vi "2HP_EnFlo_Specific - USB.vi"(5 "Datalog file path (full)":path, 6 "COM port":refnum<visa-resource-name>, 7 "Log data stream":bool, 8 "Set data rate (Hz)":u8(ring)=14 items=["1", "2", "4", "5", "8", "10", "16", "20", "25", "32", "40", "50", "64", "80", "100", "125", "160", "200", "250", "320", "400", "500", "625", "800", "1000"], 9 "N samples":u32=1000, 10 "Command":T2="s") -> (0 "Error":errorcluster, 2 "All samples out":sgl[][](array[numeric]), 3 "Rendezvous out":bool)   [LabVIEW 2020]
uses:
  ctls/2HP_Cmd (USB).ctl
  Globals/Meas_global.vi
panel:
  in  "Main":T1(tab)
  out "Serial number":u32 format="%0d"
  out "Pressure sensor EEPROM checksums ok":bool[](array[boolean])
  out "Pressure sensor temperatures in range":bool[](array[boolean])
  out "Pressure sensor values in range":bool[](array[boolean])
  out "Subsystems ok":bool[](array[boolean])
  out "n":u16
  out "Auto zero progBar":u16(slide) caption="Collecting samples, please maintain dP = 0" scale=0.0..1000.0
  out "P_raw_Azero":sgl[](array[numeric])
  in  "EEPROM array":sgl[](array[numeric])
  out "Chk ok":bool
  out "EEPROM CRC16":u16 format="%04x"
  out "received":bool
  out "Returned data rate (Hz)":u16
  out "sent":bool
  out "frm err":u32
  out "chk err":u32
  in  "Stop Data":bool
  out "Relative humidity (%)":sgl
  out "Env. sensor die temperature (deg C)":sgl
  out "External thermistor temperature (deg C)":sgl
  out "Atmospheric pressure (mbar)":sgl
  out "Checksum ok":bool
  out "Gyration vector (deg / s)":sgl[](array[numeric])
  out "Acceleration vector (g)":sgl[](array[numeric])
  out "Pressures":sgl[][](graph)
  out "Stream enabled":bool
  # "Paul Nathan 10/2020"
  # "Output array order:\nP0.... (Pa)\nP1.... (Pa)\nP_atmos (mbar)....\nT_ext (deg C)....\nT_env (deg C)....\nRH (%)....\nax (g)....\nay (g)....\naz (g)....\nwx (deg / s)....\nwy (deg / s)....\nwz (deg / s)...."
  # "Pressure sensor 0 EEPROM checksum okay"
  # "Pressure sensor 1 EEPROM checksum okay"
  # "Pressure sensor 0 temperature in range"
  # "Pressure sensor 1 temperature in range"
  # "Pressure sensor 0 value in range"
  # "Pressure sensor 1 value in range"
  # "Environmental sensor present"
  # "Inertial sensor present"
  # "Accelerometer self test pass"
  # "Gyroscope self test pass"
  # "External thermistor value in range"
  # "MCU EEPROM checksum ok"
  # "of 1000"
  # "P0 raw auto-zero"
  # "P1 raw auto-zero"
  # "P0 raw auto-zero"
  # "P1 raw auto-zero"
  # "Atmospheric pressure offset (Pa)"
  # "External thermistor temperature offset (deg C)"
  # "Serial number"
  # "RS-485 baud rate (bps)"
  # "Accelerometer vector magnitude scale factor"
  # "(reserved, 0x00000000)"
  # "(reserved, 0x00000000)"
  # "Gyroscope x component offset (deg / s)"
  # "Gyroscope y component offset (deg / s)"
  # "Gyroscope z component offset (deg / s)"
  # "RS-485 address"
  # "w_x"
  # "w_y"
  # "w_z"
  # "a_x"
  # "a_y"
  # "a_z"
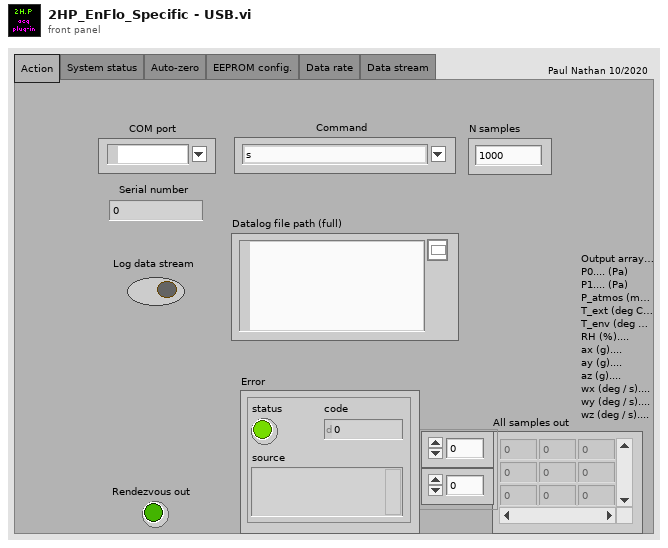
[diagram p1: front panel]
types:
  T1 = enum32{"Action", "System status", "Auto-zero", "EEPROM config.", "Data rate", "Data stream"}
  T2 = typedef "2HP_Cmd (USB).ctl" = string
  T3 = enum16{"open", "replace", "create", "open or create", "replace or create", "replace or create with confirmation"}
  T4 = typedef "Rendezvous RefNum" = refnum<k1>
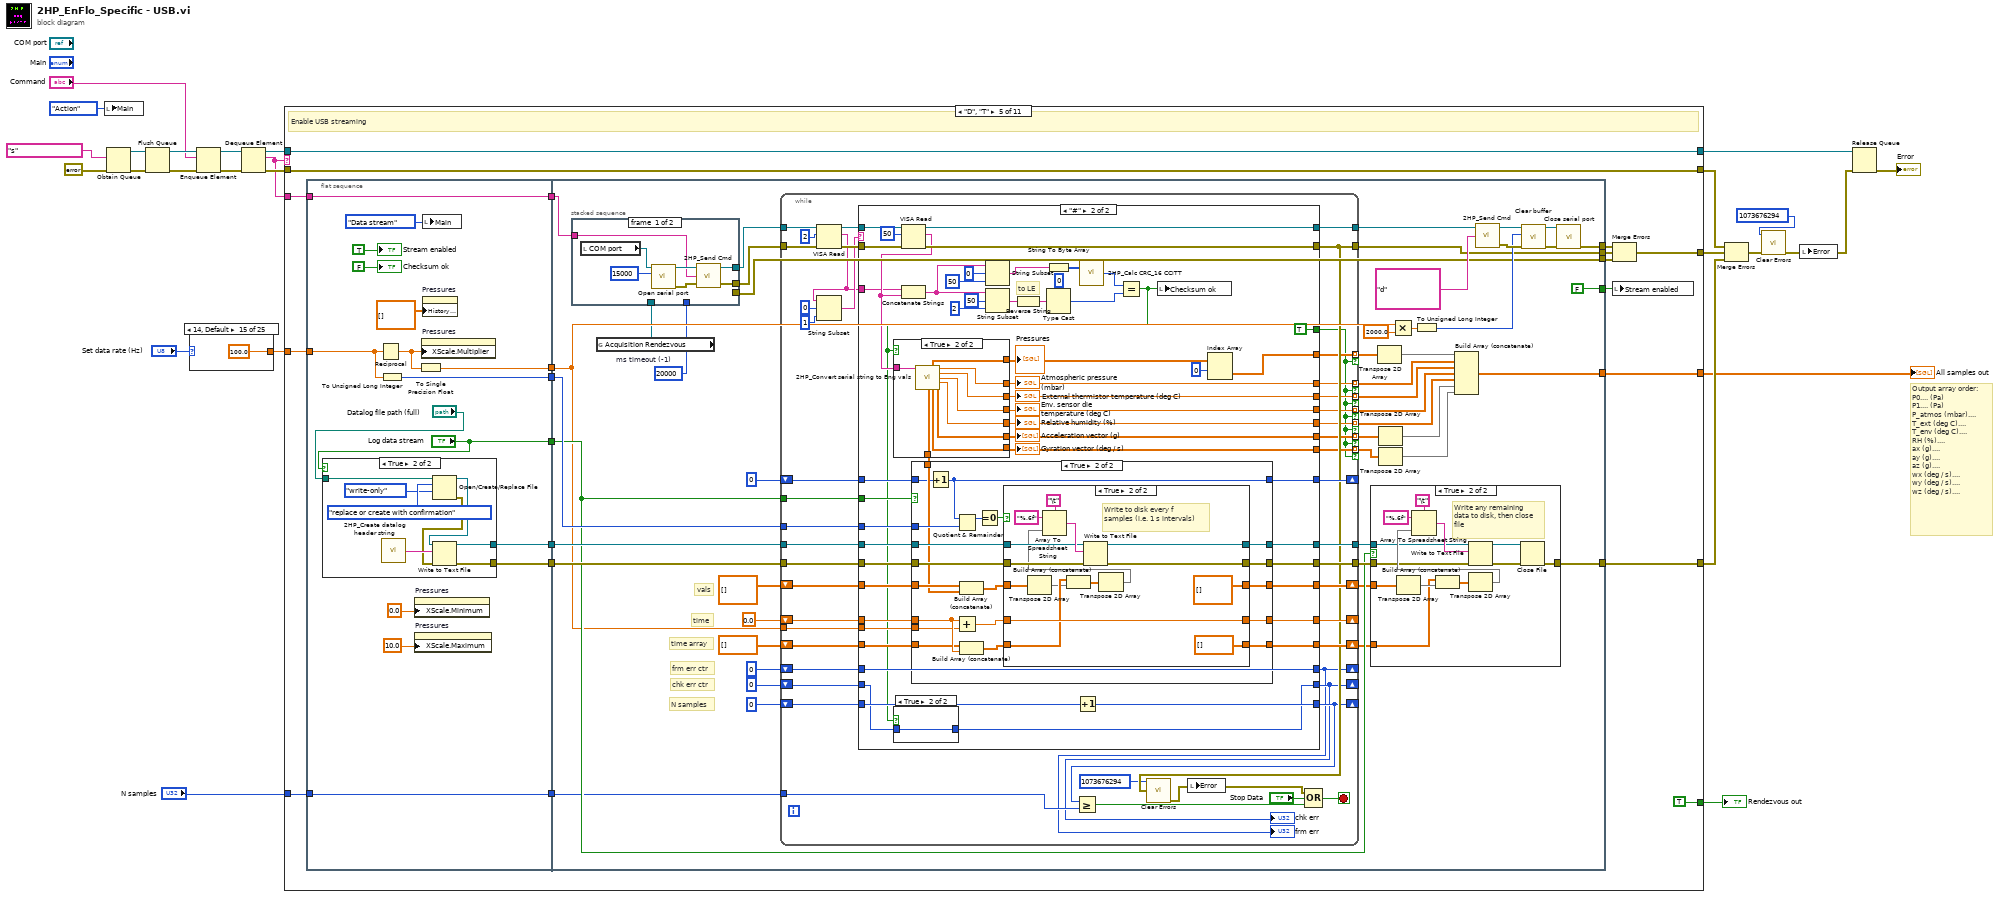
[diagram p0: block diagram]
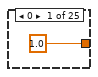
[diagram p2: hidden frame]
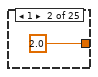
[diagram p3: hidden frame]
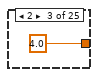
[diagram p4: hidden frame]
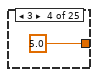
[diagram p5: hidden frame]
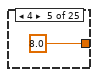
[diagram p6: hidden frame]
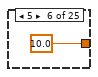
[diagram p7: hidden frame]
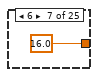
[diagram p8: hidden frame]
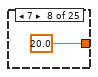
[diagram p9: hidden frame]
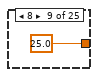
[diagram p10: hidden frame]
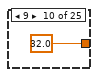
[diagram p11: hidden frame]
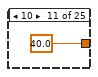
[diagram p12: hidden frame]
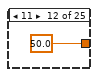
[diagram p13: hidden frame]
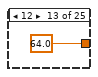
[diagram p14: hidden frame]
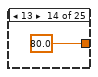
[diagram p15: hidden frame]
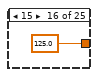
[diagram p16: hidden frame]
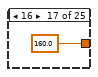
[diagram p17: hidden frame]
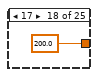
[diagram p18: hidden frame]
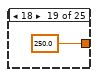
[diagram p19: hidden frame]
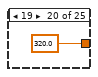
[diagram p20: hidden frame]
diagram:
  # "Output array order:\nP0.... (Pa)\nP1.... (Pa)\nP_atmos (mbar)....\nT_ext (deg C)....\nT_env (deg C)....\nRH (%)....\nax (g)....\nay (g)....\naz (g)....\nwx (deg / s)....\nwy (deg / s)....\nwz (deg / s)...."
  n1 = local write "Main"(T1."Action" ("Main")) -> ()
  n2 = Obtain Queue(element data type=T2 "s" ("Combo Box"), error in (no error)=errorcluster {"status"=FALSE, "code"=0, "source"=""}) -> (queue out=w24:refnum<queue>, error out=w25:errorcluster)  [unwired: 3 in, 1 out]
  n3 = Flush Queue(queue=w24, error in (no error)=w25) -> (queue out=w23:refnum<queue>, error out=w18:errorcluster)  [unwired: 1 out]
  n4 = case shown="14, Default" "Set data rate (Hz)" {
    tunnel: [1.0 2.0 4.0 5.0 8.0 10.0 16.0 20.0 25.0 32.0 40.0 50.0 64.0 80.0 100.0 125.0 160.0 200.0 250.0 320.0 400.0 500.0 625.0 800.0 1000.0] -> w3
    frame 0 {
    }
    frame 1 {
    }
    frame 2 {
    }
    frame 3 {
    }
    frame 4 {
    }
    frame 5 {
    }
    frame 6 {
    }
    frame 7 {
    }
    frame 8 {
    }
    frame 9 {
    }
    frame 10 {
    }
    frame 11 {
    }
    frame 12 {
    }
    frame 13 {
    }
    frame 14, Default {
    }
    frame 15 {
    }
    frame 16 {
    }
    frame 17 {
    }
    frame 18 {
    }
    frame 19 {
    }
    frame 20 {
    }
    frame 21 {
    }
    frame 22 {
    }
    frame 23 {
    }
    frame 24 {
    }
  }
  n5 = Enqueue Element(queue=w23, element="Command", error in (no error)=w18) -> (queue out=w19:refnum<queue>, error out=w17:errorcluster)  [unwired: 1 in, 1 out]
  n6 = Dequeue Element(queue=w19, error in (no error)=w17) -> (queue out=w14:refnum<queue>, element=w12:T2, error out=w13:errorcluster)  [unwired: 1 in, 1 out]
  n7 = case shown="\"D\", \"T\"" w12 {
    tunnel: w14 -> [w57 w96 w133 w183 w237 w518 w542 w596 w629 w652 w656]
    tunnel: [w57 w96 w133 w183 w237 w518 w542 w596 w629 w652 w656] -> w15
    tunnel: w13 -> [w56 w95 w132 w182 w236 w517 w543 w597 w628 w651 w655]
    tunnel: [w56 w95 w132 w182 w236 w517 w543 w597 w628 w651 w655] -> w11
    tunnel: w12 -> [w55 w94 w131 w181 w235 w520 w545 w599 w627 _ _]
    tunnel: [w53 w92 w129 w179 w220 w519 w544 w598 w625 errorcluster {"status"=FALSE, "code"=0, "source"=""} ("Error out") errorcluster {"status"=FALSE, "code"=0, "source"=""} ("Error out")] -> w10
    tunnel: [_ _ _ _ w233 _ _ _ _ _ _] -> w9
    tunnel: "N samples" -> [_ _ _ _ w226 _ _ _ _ _ _]
    tunnel: [_ _ _ _ w224 _ _ _ _ _ _] -> w5
    tunnel: w3 -> [_ _ _ _ w223 w515 _ _ _ _ _]
    tunnel: [FALSE FALSE FALSE FALSE TRUE FALSE FALSE FALSE FALSE FALSE FALSE] -> w1
    frame "S", "s" {
      # "Perform self-test and retrieve status bytes, Retrieve status bytes"
      n8 = flat-sequence {
        tunnel: w55 -> [w60]
        tunnel: [w60] -> w54
        tunnel: w54 -> [w66]
        tunnel: [w61] -> w53
        frame #0 {
          w59 = bool[] [] ("Pressure sensor EEPROM checksums ok")
          n9 = local write "Main"(T1."System status" ("Main")) -> ()
          "Pressure sensor EEPROM checksums ok" <- w59
          "Pressure sensor temperatures in range" <- w59
          "Pressure sensor values in range" <- w59
          "Subsystems ok" <- w59
        }
        frame #1 {
          w70 = 1 ("length (rest)")
          w78 = u8 0 ("byte count")
          n10 = local read "COM port"() -> (w67:refnum<visa-resource-name>)
          n11 = call "Open serial port.vi"("timeout (ms)"=u32 5000, "VISA resource name"=w67) -> ("Error out"=w88:errorcluster, "VISA resource name out"=w89:refnum<visa-resource-name>)  [unwired: 8 in]
          n12 = call "2HP_Send Cmd.vi"("Error In"=w88, "Operation"=w66, "Port"=w89) -> ("Error Out"=w86:errorcluster, "Port out"=w87:refnum<visa-resource-name>)  [unwired: 1 in]
          n13 = VISA Read(VISA resource name=w87, byte count=u32 4, error in (no error)=w86) -> (VISA resource name out=w84:refnum<visa-resource-name>, read buffer=w73:string, error out=w83:errorcluster)  [unwired: 1 out]
          n14 = call "Close serial port.vi"("Error in"=w83, "VISA resource name"=w84) -> ("Error out"=w61:errorcluster)  [unwired: 9 in]
          n15 = String Subset(string=w73, offset (0)=0, length (rest)=w70) -> (substring=w82:string)
          n16 = String Subset(string=w73, offset (0)=1, length (rest)=w70) -> (substring=w81:string)
          n17 = String Subset(string=w73, offset (0)=2 ("length (rest)"), length (rest)=w70) -> (substring=w80:string)
          n18 = String Subset(string=w73, offset (0)=3, length (rest)=w70) -> (substring=w79:string)
          n19 = Type Cast(type=w78, x=w82) -> (*(type *) &x=w77:u8)
          n20 = Type Cast(type=w78, x=w81) -> (*(type *) &x=w76:u8)
          n21 = Type Cast(type=w78, x=w80) -> (*(type *) &x=w75:u8)
          n22 = Type Cast(type=w78, x=w79) -> (*(type *) &x=w74:u8)
          n23 = Number To Boolean Array(number=w77) -> (Boolean array=w65:bool[])
          n24 = Number To Boolean Array(number=w76) -> (Boolean array=w64:bool[])
          n25 = Number To Boolean Array(number=w75) -> (Boolean array=w63:bool[])
          n26 = Number To Boolean Array(number=w74) -> (Boolean array=w62:bool[])
          n27 = local write "Pressure sensor EEPROM checksums ok"(w65) -> ()
          n28 = local write "Pressure sensor temperatures in range"(w64) -> ()
          n29 = local write "Pressure sensor values in range"(w63) -> ()
          n30 = local write "Subsystems ok"(w62) -> ()
        }
      }
    }
    frame "Z", "z" {
      # "Perform permanent auto-zero (write values to EEPROM), Perform temporary auto-zero"
      n31 = flat-sequence {
        tunnel: w94 -> [w100]
        tunnel: [w100] -> w93
        tunnel: w93 -> [w107]
        tunnel: [w103] -> w92
        frame #0 {
          n32 = local write "Main"(T1."Auto-zero" ("Main")) -> ()
          "P_raw_Azero" <- sgl[] [] ("P_raw_Azero")
          "Auto zero progBar" <- u16 0 ("Collecting samples, please maintain dP = 0")
        }
        frame #1 {
          n33 = local read "COM port"() -> (w108:refnum<visa-resource-name>)
          n34 = call "Open serial port.vi"("timeout (ms)"=u32 16000, "VISA resource name"=w108) -> ("Error out"=w114:errorcluster, "VISA resource name out"=w115:refnum<visa-resource-name>)  [unwired: 8 in]
          n35 = call "2HP_Send Cmd.vi"("Error In"=w114, "Operation"=w107, "Port"=w115) -> ("Error Out"=w112:errorcluster, "Port out"=w113:refnum<visa-resource-name>)  [unwired: 1 in]
          n36 = VISA Read(VISA resource name=w113, byte count=u32 8, error in (no error)=w112) -> (VISA resource name out=w110:refnum<visa-resource-name>, read buffer=w104:string, error out=w109:errorcluster)  [unwired: 1 out]
          n37 = for {
            N: 1000 -> [_]
            shift-right: [w117] -> _
            shift-left: u16 0 -> [w118]
            n38 = Increment(x=w118) -> (x+1=w117:u16)
            "n" <- w117
            n39 = Wait (ms)(milliseconds to wait=u32 11) -> ()  [unwired: 1 out]
            n40 = local write "Auto zero progBar"(w117) -> ()
          }
          n41 = for {
            N: 2 -> [_]
            tunnel: [w121] -> w106 mode=indexing
            tunnel: w104 -> [w120]
            i -> [w127]
            w125 = 4 ("x")
            # "to BE"
            n42 = Multiply(x=w125, y=w127) -> (x*y=w126:i32)
            n43 = String Subset(string=w120, offset (0)=w126, length (rest)=w125) -> (substring=w124:string)
            n44 = Reverse String(1:w124) -> (0:w123:string)
            n45 = Type Cast(type=sgl 0.0 ("byte count"), x=w123) -> (*(type *) &x=w121:sgl)
          }
          n46 = call "Close serial port.vi"("Error in"=w109, "VISA resource name"=w110) -> ("Error out"=w103:errorcluster)  [unwired: 9 in]
          n47 = local write "P_raw_Azero"(w106) -> ()
        }
      }
    }
    frame "R" {
      # "Read all EEPROM values"
      n48 = flat-sequence {
        tunnel: w131 -> [w136]
        tunnel: [w136] -> w130
        tunnel: w130 -> [w159]
        tunnel: [w158] -> w129
        frame #0 {
          n49 = local write "Main"(T1."EEPROM config." ("Main")) -> ()
          n50 = local write "EEPROM array"(sgl[] [] ("EEPROM array")) -> ()
        }
        frame #1 {
          (unwired) 1 ("length (rest)")
          # "to BE"
          n51 = local read "COM port"() -> (w160:refnum<visa-resource-name>)
          n52 = call "Open serial port.vi"("timeout (ms)"=u32 5000, "VISA resource name"=w160) -> ("Error out"=w166:errorcluster, "VISA resource name out"=w167:refnum<visa-resource-name>)  [unwired: 8 in]
          n53 = call "2HP_Send Cmd.vi"("Error In"=w166, "Operation"=w159, "Port"=w167) -> ("Error Out"=w164:errorcluster, "Port out"=w165:refnum<visa-resource-name>)  [unwired: 1 in]
          n54 = VISA Read(VISA resource name=w165, byte count=u32 51, error in (no error)=w164) -> (VISA resource name out=w162:refnum<visa-resource-name>, read buffer=w138:string, error out=w161:errorcluster)  [unwired: 1 out]
          n55 = call "Close serial port.vi"("Error in"=w161, "VISA resource name"=w162) -> ("Error out"=w158:errorcluster)  [unwired: 9 in]
          n56 = String Subset(string=w138, offset (0)=48) -> (substring=w142:string)  [unwired: 1 in]
          n57 = String Subset(string=w138, offset (0)=49, length (rest)=2 ("length (rest)")) -> (substring=w154:string)
          n58 = String Subset(string=w138, offset (0)=0, length (rest)=49 ("length (rest)")) -> (substring=w157:string)
          n59 = for {
            N: 12 -> [_]
            tunnel: [w172] -> w147 mode=indexing
            tunnel: w138 -> [w171]
            i -> [w176]
            w174 = 4 ("x")
            # "to BE"
            n60 = Multiply(x=w174, y=w176) -> (x*y=w175:i32)
            n61 = String Subset(string=w171, offset (0)=w175, length (rest)=w174) -> (substring=w170:string)
            n62 = Reverse String(1:w170) -> (0:w169:string)
            n63 = Type Cast(type=sgl 0.0 ("byte count"), x=w169) -> (*(type *) &x=w172:sgl)
          }
          n64 = Reverse String(1:w154) -> (0:w150:string)
          n65 = String To Byte Array(string=w157) -> (unsigned byte array=w148:u8[])
          n66 = Type Cast(type=u8 0 ("byte count"), x=w142) -> (*(type *) &x=w141:u8)
          n67 = call "2HP_Calc CRC_16 CCITT.vi"("Data bytes"=w148) -> ("CRC_16-CCITT"=w149:u16)  [unwired: 1 in]
          n68 = Type Cast(type=u16 0 ("byte count"), x=w150) -> (*(type *) &x=w145:u16)
          n69 = To Single Precision Float(number=w141) -> (single precision float=w137:sgl)
          n70 = Equal?(x=w145, y=w149) -> (x = y?=w144:bool)
          n71 = Build Array (concatenate)(w147, w137) -> (w143:sgl[])
          n72 = local write "EEPROM array"(w143) -> ()
          n73 = local write "EEPROM CRC16"(w145) -> ()
          n74 = local write "Chk ok"(w144) -> ()
        }
      }
    }
    frame "W" {
      # "Write all EEPROM values (including new checksum)"
      n75 = flat-sequence {
        tunnel: w181 -> [w186]
        tunnel: [w186] -> w180
        tunnel: ["EEPROM array"] -> w177
        tunnel: w180 -> [w207]
        tunnel: [w206] -> w179
        tunnel: w177 -> [w187]
        frame #0 {
          n76 = local write "Main"(T1."EEPROM config." ("Main")) -> ()
        }
        frame #1 {
          # "to LE"
          n77 = local read "COM port"() -> (w208:refnum<visa-resource-name>)
          n78 = for {
            N: 12 -> [_]
            tunnel: w187 -> [w214] mode=indexing
            shift-right: [w215] -> w198
            shift-left: "" -> [w216]
            # "to LE"
            n79 = Type Cast(type="", x=w214) -> (*(type *) &x=w213:string)
            n80 = Reverse String(1:w213) -> (0:w212:string)
            n81 = Concatenate Strings(w216, w212) -> (w215:string)
          }
          n82 = call "Open serial port.vi"("timeout (ms)"=u32 5000, "VISA resource name"=w208) -> ("Error out"=w209:errorcluster, "VISA resource name out"=w210:refnum<visa-resource-name>)  [unwired: 8 in]
          n83 = Index Array(array=w187, index=12) -> (element=w191:sgl)
          n84 = To Unsigned Byte Integer(number=w191) -> (unsigned 8bit integer=w192:u8)
          n85 = Type Cast(type="", x=w192) -> (*(type *) &x=w188:string)
          n86 = Concatenate Strings(w198, w188) -> (w199:string)
          n87 = String To Byte Array(string=w199) -> (unsigned byte array=w200:u8[])
          n88 = call "2HP_Calc CRC_16 CCITT.vi"("Data bytes"=w200) -> ("CRC_16-CCITT"=w193:u16)  [unwired: 1 in]
          "EEPROM CRC16" <- w193
          n89 = Type Cast(type="", x=w193) -> (*(type *) &x=w201:string)
          n90 = Reverse String(1:w201) -> (0:w202:string)
          n91 = Concatenate Strings(w199, w202) -> (w194:string)
          n92 = call "7HP_Send Cmd + Data.vi"("Error In"=w209, "Data"=w194, "Operation"=w207, "Port"=w210) -> ("Error Out"=w205:errorcluster, "Port out"=w204:refnum<visa-resource-name>)  [unwired: 1 in]
          n93 = call "Close serial port.vi"("Error in"=w205, "VISA resource name"=w204) -> ("Error out"=w206:errorcluster)  [unwired: 9 in]
          "Chk ok" <- TRUE ("Chk ok")
        }
      }
    }
    frame "D", "T" {
      # "Enable USB streaming"
      n94 = flat-sequence {
        tunnel: w235 -> [w253]
        tunnel: [w253] -> w234
        tunnel: [w250] -> w232
        tunnel: [w249] -> w231
        tunnel: [w247] -> w230
        tunnel: w223 -> [w248]
        tunnel: [w245] -> w229
        tunnel: ["Log data stream"] -> w228
        tunnel: w226 -> [w241]
        tunnel: [w241] -> w225
        tunnel: w234 -> [w271]
        tunnel: [w310] -> w221
        tunnel: [w309] -> w233
        tunnel: w232 -> [w306]
        tunnel: w231 -> [w305]
        tunnel: w230 -> [w307]
        tunnel: w229 -> [w273]
        tunnel: w228 -> [w299]
        tunnel: [FALSE] -> w227
        tunnel: w225 -> [w286]
        tunnel: [w275] -> w224
        tunnel: [w272] -> w222
        tunnel: [w268] -> w219
        frame #0 {
          n95 = case shown="True" "Log data stream" {
            tunnel: "Datalog file path (full)" -> [_ w263]
            tunnel: [refnum<file> refnum ("refnum out") w257] -> w250
            tunnel: [errorcluster {"status"=FALSE, "code"=0, "source"=""} ("error out") w256] -> w249
            frame False {
            }
            frame True {
              n96 = call "2HP_Create datalog header string.vi"() -> ("Datalog header string"=w259:string)  [unwired: 1 in]
              n97 = Open/Create/Replace File(file path (use dialog)=w263, operation (0:open)=T3."replace or create with confirmation", access (0:read/write)=enum16{"read/write", "read-only", "write-only"}."write-only") -> (refnum out=w260:refnum<file>, error out=w258:errorcluster)  [unwired: 3 in, 1 out]
              n98 = Write to Text File(file (use dialog)=w260, text=w259, error in=w258) -> (refnum out=w257:refnum<file>, error out=w256:errorcluster)  [unwired: 1 in, 1 out]
            }
          }
          n99 = Reciprocal(x=w248) -> (1/x=w246:dbl)
          n100 = To Unsigned Long Integer(number=w248) -> (unsigned 32bit integer=w247:u32)
          n101 = property on="Pressures" class="WFChart (strict)"("XScale.Minimum"=0.0 ("X Scale.Range:Minimum")) -> ()  [unwired: 2 in, 2 out]
          n102 = property on="Pressures" class="WFChart (strict)"("XScale.Maximum"=10.0 ("X Scale.Range:Maximum")) -> ()  [unwired: 2 in, 2 out]
          n103 = To Single Precision Float(number=w246) -> (single precision float=w245:sgl)
          n104 = property on="Pressures" class="WFChart (strict)"("XScale.Multiplier"=w246) -> ()  [unwired: 2 in, 2 out]
          n105 = local write "Main"(T1."Data stream" ("Main")) -> ()
          n106 = property on="Pressures" class="WFChart (strict)"("History Data"=sgl[][] []) -> ()  [unwired: 2 in, 2 out]
          "Checksum ok" <- FALSE ("Checksum ok")
          "Stream enabled" <- TRUE ("Stream enabled")
        }
        frame #1 {
          w266 = 20000  # ms timeout (-1)
          # "N samples"
          # "chk err ctr"
          # "frm err ctr"
          # "vals"
          # "time"
          # "time array"
          n107 = global read "Meas_global.vi" "Acquisition Rendezvous"() -> (w267:T4)
          n108 = stacked-sequence {
            tunnel: w271 -> [w314 _]
            tunnel: [w311 _] -> w269
            tunnel: [w312 _] -> w270
            tunnel: [_ w320] -> w268
            tunnel: w267 -> [_ w319]
            tunnel: w266 -> [_ w318]
            frame #0 {
              n109 = local read "COM port"() -> (w316:refnum<visa-resource-name>)
              n110 = call "Open serial port.vi"("timeout (ms)"=u32 15000, "VISA resource name"=w316) -> ("Error out"=w313:errorcluster, "VISA resource name out"=w315:refnum<visa-resource-name>)  [unwired: 8 in]
              n111 = call "2HP_Send Cmd.vi"("Error In"=w313, "Operation"=w314, "Port"=w315) -> ("Error Out"=w311:errorcluster, "Port out"=w312:refnum<visa-resource-name>)  [unwired: 1 in]
            }
            frame #1 {
              # "Wait here until all acq. devs. are ready."
              n112 = call <vilib>:"Wait at Rendezvous.vi"("ms timeout (-1)"=w318, "rendezvous"=w319) -> ("error out"=w320:errorcluster)  [unwired: 3 in, 2 out]
            }
          }
          n113 = while {
            tunnel: [w358] -> w272
            tunnel: w270 -> [w359]
            tunnel: [w377] -> w298
            shift-right: [w373] -> _
            shift-left: u32 0 -> [w374]
            tunnel: w307 -> [w372]
            tunnel: w306 -> [w371]
            tunnel: w305 -> [w370]
            tunnel: [w369] -> w304
            tunnel: [w368] -> w303
            shift-right: [w367] -> w289
            shift-left: sgl[][] [] -> [w366]
            shift-right: [w363] -> _
            shift-left: sgl 0.0 ("Numeric") -> [w365]
            tunnel: w273 -> [w364]
            shift-right: [w361] -> w288
            shift-left: sgl[] [] -> [w362]
            tunnel: w299 -> [w360]
            shift-right: [w352] -> _
            shift-left: u32 0 -> [w355]
            tunnel: w286 -> [w354]
            tunnel: [w351] -> w285 mode=indexing if=w344
            tunnel: [w350] -> w281 mode=indexing if=w344
            tunnel: [w349] -> w280 mode=indexing if=w344
            tunnel: [w348] -> w279 mode=indexing if=w344
            tunnel: [w347] -> w278 mode=indexing if=w344
            tunnel: [w346] -> w283 mode=indexing if=w344
            tunnel: [w345] -> w282 mode=indexing if=w344
            tunnel: w269 -> [w343]
            shift-right: [w339] -> _
            shift-left: u32 0 -> [w341]
            shift-right: [w340] -> _
            shift-left: u32 0 -> [w342]
            stop <- w375 stop-if-true
            n114 = VISA Read(VISA resource name=w359, byte count=u32 2, error in (no error)=w343) -> (VISA resource name out=w379:refnum<visa-resource-name>, read buffer=w335:string, error out=w378:errorcluster)  [unwired: 1 out]
            n115 = String Subset(string=w335, offset (0)=0, length (rest)=1 ("length (rest)")) -> (substring=w336:string)
            n116 = case shown="\"#\"" w336 {
              tunnel: w379 -> [w392 w443]
              tunnel: [w393 w441] -> w358
              tunnel: w378 -> [w393 w444]
              tunnel: [w392 w442] -> w377
              tunnel: w374 -> [w391 w413]
              tunnel: [w391 w399] -> w373
              tunnel: w372 -> [_ w411]
              tunnel: w371 -> [w390 w410]
              tunnel: w370 -> [w389 w409]
              tunnel: [w389 w401] -> w369
              tunnel: [w390 w400] -> w368
              tunnel: [w388 w402] -> w367
              tunnel: w366 -> [w388 w408]
              tunnel: w365 -> [w387 w407]
              tunnel: w364 -> [_ w406]
              tunnel: [w387 w403] -> w363
              tunnel: w362 -> [w386 w405]
              tunnel: [w386 w404] -> w361
              tunnel: w360 -> [_ w412]
              tunnel: w355 -> [w385 w439]
              tunnel: [w385 w438] -> w352
              tunnel: [_ w437] -> w351
              tunnel: [FALSE TRUE] -> w344
              tunnel: [_ w436] -> w350
              tunnel: [_ w435] -> w349
              tunnel: [_ w434] -> w348
              tunnel: [_ w433] -> w347
              tunnel: [_ w432] -> w346
              tunnel: [_ w431] -> w345
              tunnel: w342 -> [w381 w396]
              tunnel: w341 -> [w383 w398]
              tunnel: [w382 w398] -> w339
              tunnel: [w381 w395] -> w340
              tunnel: w335 -> [_ w394]
              frame Default {
                n117 = Increment(x=w383) -> (x+1=w382:u32)
              }
              frame "#" {
                # "to LE"
                n118 = VISA Read(VISA resource name=w443, byte count=u32 50, error in (no error)=w444) -> (VISA resource name out=w442:refnum<visa-resource-name>, read buffer=w428:string, error out=w441:errorcluster)  [unwired: 1 out]
                n119 = Concatenate Strings(w394, w428) -> (w417:string)
                n120 = String Subset(string=w417, offset (0)=0, length (rest)=50 ("length (rest)")) -> (substring=w423:string)
                n121 = String Subset(string=w417, offset (0)=50, length (rest)=2 ("length (rest)")) -> (substring=w426:string)
                n122 = Reverse String(1:w426) -> (0:w425:string)
                n123 = String To Byte Array(string=w423) -> (unsigned byte array=w416:u8[])
                n124 = Type Cast(type=u16 0 ("length (rest)"), x=w425) -> (*(type *) &x=w424:u16)
                n125 = Increment(x=w439) -> (x+1=w438:u32)
                n126 = call "2HP_Calc CRC_16 CCITT.vi"("Data bytes"=w416) -> ("CRC_16-CCITT"=w415:u16)  [unwired: 1 in]
                n127 = Equal?(x=w415, y=w424) -> (x = y?=w397:bool)
                n128 = case shown="True" w397 {
                  tunnel: [w504 w506] -> w436
                  tunnel: [w504 w505] -> w435
                  tunnel: [w504 w513] -> w434
                  tunnel: [w504 w512] -> w433
                  tunnel: [w497 w511] -> w432
                  tunnel: [w497 w510] -> w431
                  tunnel: [w495 w509] -> w414
                  tunnel: [w503 w508] -> w430
                  tunnel: w428 -> [_ w507]
                  frame False {
                    w504 = sgl nan ("Atmospheric pressure (mbar)")
                    n129 = Initialize Array(sgl nan ("element"), 2 ("dimension size")) -> (w502:sgl[])
                    n130 = Initialize Array(sgl nan ("element"), 3 ("dimension size")) -> (w497:sgl[])
                    n131 = Initialize Array(sgl nan ("element"), 12 ("dimension size")) -> (w495:sgl[])
                    n132 = Build Array(w502) -> (w503:sgl[][])
                  }
                  frame True {
                    n133 = call "2HP_Convert serial string to Eng vals.vi"("Serial buffer string (excluding FrameChar)"=w507) -> ("Pressures"=w508:sgl[][], "Atmospheric pressure (mbar)"=w506:sgl, "External thermistor temperature (deg C)"=w505:sgl, "Env. sensor die temperature (deg C)"=w513:sgl, "Relative humidity (%)"=w512:sgl, "All vals"=w509:sgl[], "Gyration vector (deg / s)"=w510:sgl[], "Acceleration vector (g)"=w511:sgl[])  [unwired: 7 in]
                  }
                }
                "Pressures" <- w430
                "Acceleration vector (g)" <- w432
                "Gyration vector (deg / s)" <- w431
                "Atmospheric pressure (mbar)" <- w436
                "External thermistor temperature (deg C)" <- w435
                "Env. sensor die temperature (deg C)" <- w434
                "Relative humidity (%)" <- w433
                n134 = case shown="True" w397 {
                  tunnel: w396 -> [w446 w447]
                  tunnel: [w445 w447] -> w395
                  frame False {
                    n135 = Increment(x=w446) -> (x+1=w445:u32)
                  }
                  frame True {
                  }
                }
                n136 = case shown="True" w412 {
                  tunnel: w413 -> [w453 w455]
                  tunnel: [w453 w454] -> w399
                  tunnel: w411 -> [_ w473]
                  tunnel: w414 -> [_ w459]
                  tunnel: w410 -> [w451 w470]
                  tunnel: w409 -> [w452 w469]
                  tunnel: [w452 w468] -> w401
                  tunnel: [w451 w467] -> w400
                  tunnel: w408 -> [w450 w460]
                  tunnel: [w450 w466] -> w402
                  tunnel: w407 -> [w449 w463]
                  tunnel: w406 -> [_ w462]
                  tunnel: [w449 w465] -> w403
                  tunnel: w405 -> [w448 w461]
                  tunnel: [w448 w464] -> w404
                  frame False {
                  }
                  frame True {
                    n137 = Increment(x=w455) -> (x+1=w454:u32)
                    n138 = Add(x=w463, y=w462) -> (x+y=w458:sgl)
                    n139 = Quotient & Remainder(x=w454, y=w473) -> (x-y*floor(x/y)=w472:u32)  [unwired: 1 out]
                    n140 = Build Array (concatenate)(w460, w459) -> (w456:sgl[][])
                    n141 = Build Array (concatenate)(w461, w463) -> (w457:sgl[])
                    n142 = Equal To 0?(x=w472) -> (x = 0?=w471:bool)
                    n143 = case shown="True" w471 {
                      tunnel: w470 -> [w477 w490]
                      tunnel: w469 -> [w478 w489]
                      tunnel: [w478 w488] -> w468
                      tunnel: [w477 w487] -> w467
                      tunnel: w456 -> [w475 w482]
                      tunnel: [w475 sgl[][] []] -> w466
                      tunnel: w458 -> [w476 w485]
                      tunnel: [w476 w485] -> w465
                      tunnel: w457 -> [w474 w484]
                      tunnel: [w474 sgl[] []] -> w464
                      frame False {
                      }
                      frame True {
                        # "Write to disk every f samples (i.e. 1 s intervals)"
                        n144 = Transpose 2D Array(2D array=w482) -> (transposed array=w481:sgl[][])
                        n145 = Build Array (concatenate)(w484, w481) -> (w480:sgl[][])
                        n146 = Transpose 2D Array(2D array=w480) -> (transposed array=w479:sgl[][])
                        n147 = Array To Spreadsheet String(delimiter (Tab)="\t", array=w479, 3:"%.6f" ("format string")) -> (spreadsheet string=w493:string)
                        n148 = Write to Text File(file (use dialog)=w490, text=w493, error in=w489) -> (refnum out=w487:refnum<file>, error out=w488:errorcluster)  [unwired: 1 in, 1 out]
                      }
                    }
                  }
                }
                n149 = local write "Checksum ok"(w397) -> ()
                n150 = Index Array(array=w430, index (row)=0) -> (element=w437:sgl[])  [unwired: 1 in]
              }
            }
            "chk err" <- w340
            "frm err" <- w339
            n151 = Greater Or Equal?(x=w352, y=w354) -> (x >= y?=w353:bool)
            n152 = call <vilib>:"Clear Errors.vi"("error in (no error)"=w358, "specific error code to clear (0: all)"=1073676294) -> ("error out"=w357:errorcluster)  [unwired: 4 in, 1 out]
            n153 = local write "Error"(w357) -> ()
            n154 = Compound Arithmetic op=OR(w357, "Stop Data", w353) -> (w375:bool)
          }
          n155 = case shown="True" w299 {
            tunnel: [w321 w334] -> w309
            tunnel: w304 -> [w321 w326]
            tunnel: w303 -> [_ w327]
            tunnel: w289 -> [_ w325]
            tunnel: w288 -> [_ w324]
            frame False {
            }
            frame True {
              # "Write any remaining data to disk, then close file"
              n156 = Transpose 2D Array(2D array=w325) -> (transposed array=w331:sgl[][])
              n157 = Build Array (concatenate)(w324, w331) -> (w332:sgl[][])
              n158 = Transpose 2D Array(2D array=w332) -> (transposed array=w333:sgl[][])
              n159 = Array To Spreadsheet String(delimiter (Tab)="\t", array=w333, 3:"%.6f" ("format string")) -> (spreadsheet string=w328:string)
              n160 = Write to Text File(file (use dialog)=w327, text=w328, error in=w326) -> (refnum out=w323:refnum<file>, error out=w322:errorcluster)  [unwired: 1 in, 1 out]
              n161 = Close File(refnum=w323, error in=w322) -> (error out=w334:errorcluster)  [unwired: 1 out]
            }
          }
          n162 = Transpose 2D Array(2D array=w285) -> (transposed array=w284:sgl[][])
          n163 = Transpose 2D Array(2D array=w283) -> (transposed array=w277:sgl[][])
          n164 = Transpose 2D Array(2D array=w282) -> (transposed array=w276:sgl[][])
          n165 = Multiply(x=w273, y=sgl 2000.0) -> (x*y=w292:sgl)
          n166 = To Unsigned Long Integer(number=w292) -> (unsigned 32bit integer=w290:u32)
          n167 = Build Array (concatenate)(w284, w281, w280, w279, w278, w277, w276) -> (w275:sgl[][])
          n168 = call "2HP_Send Cmd.vi"("Operation"=T2 "d" ("Combo Box"), "Port"=w298) -> ("Error Out"=w295:errorcluster, "Port out"=w296:refnum<visa-resource-name>)  [unwired: 2 in]
          n169 = call "Clear buffer.vi"("Error in"=w295, "dt for timeout (ms)"=w290, "VISA resource name in"=w296) -> ("Error out"=w293:errorcluster, "VISA resource name out"=w294:refnum<visa-resource-name>)  [unwired: 3 in]
          n170 = call "Close serial port.vi"("Error in"=w293, "VISA resource name"=w294) -> ("Error out"=w310:errorcluster)  [unwired: 9 in]
        }
      }
      n171 = Merge Errors(w221, w222, w219) -> (w220:errorcluster)
      n172 = local write "Stream enabled"(w227) -> ()
    }
    frame "d", "t" {
      # "Disable USB streaming"
      n173 = flat-sequence {
        tunnel: [w528] -> w521
        tunnel: w520 -> [w528]
        tunnel: w515 -> [w523]
        tunnel: [w522] -> w516
        tunnel: w521 -> [w536]
        tunnel: [w535] -> w519
        tunnel: w516 -> [w530]
        frame #0 {
          n174 = disable-structure shown="Disabled" {
            frame Disabled {
              n175 = local write "Main"(T1."Data stream" ("Main")) -> ()
            }
            frame Enabled {
            }
          }
          n176 = Reciprocal(x=w523) -> (1/x=w527:dbl)
          n177 = To Single Precision Float(number=w527) -> (single precision float=w525:sgl)
          n178 = Multiply(x=w525, y=sgl 2000.0) -> (x*y=w526:sgl)
          n179 = To Unsigned Long Integer(number=w526) -> (unsigned 32bit integer=w522:u32)
        }
        frame #1 {
          n180 = local read "COM port"() -> (w537:refnum<visa-resource-name>)
          n181 = call "Open serial port.vi"("timeout (ms)"=u32 5000, "VISA resource name"=w537) -> ("Error out"=w538:errorcluster, "VISA resource name out"=w539:refnum<visa-resource-name>)  [unwired: 8 in]
          n182 = call "2HP_Send Cmd.vi"("Error In"=w538, "Operation"=w536, "Port"=w539) -> ("Error Out"=w532:errorcluster, "Port out"=w534:refnum<visa-resource-name>)  [unwired: 1 in]
          n183 = call "Clear buffer.vi"("Error in"=w532, "dt for timeout (ms)"=w530, "VISA resource name in"=w534) -> ("Error out"=w531:errorcluster, "VISA resource name out"=w533:refnum<visa-resource-name>)  [unwired: 3 in]
          n184 = call "Close serial port.vi"("Error in"=w531, "VISA resource name"=w533) -> ("Error out"=w535:errorcluster)  [unwired: 9 in]
        }
      }
    }
    frame "F" {
      # "Set data rate"
      n185 = flat-sequence {
        tunnel: [w552] -> w546
        tunnel: w545 -> [w552]
        tunnel: [w559] -> w547
        tunnel: w546 -> [w557]
        tunnel: w547 -> [w593]
        tunnel: [w593] -> w544
        frame #0 {
          n186 = local write "Returned data rate (Hz)"(u16 0 ("Returned data rate (Hz)")) -> ()
          n187 = local write "received"(FALSE ("received")) -> ()
          n188 = local write "Main"(T1."Data rate" ("Main")) -> ()
          n189 = local write "sent"(FALSE ("sent")) -> ()
        }
        frame #1 {
          # "to LE"
          n190 = local read "Set data rate (Hz)"() -> (w555:u8)
          n191 = case shown="14, Default" w555 {
            tunnel: [1.0 2.0 4.0 5.0 8.0 10.0 16.0 20.0 25.0 32.0 40.0 50.0 64.0 80.0 100.0 125.0 160.0 200.0 250.0 320.0 400.0 500.0 625.0 800.0 1000.0] -> w554
            frame 0 {
            }
            frame 1 {
            }
            frame 2 {
            }
            frame 3 {
            }
            frame 4 {
            }
            frame 5 {
            }
            frame 6 {
            }
            frame 7 {
            }
            frame 8 {
            }
            frame 9 {
            }
            frame 10 {
            }
            frame 11 {
            }
            frame 12 {
            }
            frame 13 {
            }
            frame 14, Default {
            }
            frame 15 {
            }
            frame 16 {
            }
            frame 17 {
            }
            frame 18 {
            }
            frame 19 {
            }
            frame 20 {
            }
            frame 21 {
            }
            frame 22 {
            }
            frame 23 {
            }
            frame 24 {
            }
          }
          n192 = local read "COM port"() -> (w558:refnum<visa-resource-name>)
          n193 = To Unsigned Word Integer(number=w554) -> (unsigned 16bit integer=w561:u16)
          n194 = call "Open serial port.vi"("timeout (ms)"=u32 5000, "VISA resource name"=w558) -> ("Error out"=w564:errorcluster, "VISA resource name out"=w563:refnum<visa-resource-name>)  [unwired: 8 in]
          n195 = Type Cast(type="", x=w561) -> (*(type *) &x=w560:string)
          n196 = Reverse String(1:w560) -> (0:w556:string)
          n197 = call "7HP_Send Cmd + Data.vi"("Error In"=w564, "Data"=w556, "Operation"=w557, "Port"=w563) -> ("Error Out"=w566:errorcluster, "Port out"=w565:refnum<visa-resource-name>)  [unwired: 1 in]
          n198 = call "Close serial port.vi"("Error in"=w566, "VISA resource name"=w565) -> ("Error out"=w559:errorcluster)  [unwired: 9 in]
        }
        frame #2 {
          n199 = Unbundle By Name(w593) -> ("status"=w594:bool)
          n200 = Not(x=w594) -> (.not. x?=→"sent":bool)
        }
      }
    }
    frame "f" {
      # "Get data rate"
      n201 = flat-sequence {
        tunnel: [w605] -> w600
        tunnel: w599 -> [w605]
        tunnel: [w617] -> w601
        tunnel: w600 -> [w615]
        tunnel: w601 -> [w622]
        tunnel: [w622] -> w598
        frame #0 {
          n202 = local write "received"(FALSE ("received")) -> ()
          n203 = local write "Main"(T1."Data rate" ("Main")) -> ()
          n204 = local write "sent"(FALSE ("sent")) -> ()
        }
        frame #1 {
          # "to BE"
          n205 = local read "COM port"() -> (w616:refnum<visa-resource-name>)
          n206 = call "Open serial port.vi"("timeout (ms)"=u32 5000, "VISA resource name"=w616) -> ("Error out"=w620:errorcluster, "VISA resource name out"=w619:refnum<visa-resource-name>)  [unwired: 8 in]
          n207 = call "2HP_Send Cmd.vi"("Error In"=w620, "Operation"=w615, "Port"=w619) -> ("Error Out"=w609:errorcluster, "Port out"=w610:refnum<visa-resource-name>)  [unwired: 1 in]
          n208 = VISA Read(VISA resource name=w610, byte count=u32 2, error in (no error)=w609) -> (VISA resource name out=w607:refnum<visa-resource-name>, read buffer=w613:string, error out=w608:errorcluster)  [unwired: 1 out]
          n209 = Reverse String(1:w613) -> (0:w611:string)
          n210 = call "Close serial port.vi"("Error in"=w608, "VISA resource name"=w607) -> ("Error out"=w617:errorcluster)  [unwired: 9 in]
          n211 = Type Cast(type=u16 0 ("byte count"), x=w611) -> (*(type *) &x=→"Returned data rate (Hz)":u16)
        }
        frame #2 {
          n212 = Unbundle By Name(w622) -> ("status"=w623:bool)
          n213 = Not(x=w623) -> (.not. x?=→"received":bool)
        }
      }
    }
    frame "N" {
      # "Get serial number"
      n214 = flat-sequence {
        tunnel: w627 -> [w632]
        tunnel: [w632] -> w626
        tunnel: w626 -> [w639]
        tunnel: [w638] -> w625
        frame #0 {
          n215 = local write "Main"(T1."Action" ("Main")) -> ()
          "Serial number" <- u32 0 ("Numeric")
        }
        frame #1 {
          # "to BE"
          n216 = local read "COM port"() -> (w640:refnum<visa-resource-name>)
          n217 = call "Open serial port.vi"("timeout (ms)"=u32 5000, "VISA resource name"=w640) -> ("Error out"=w646:errorcluster, "VISA resource name out"=w647:refnum<visa-resource-name>)  [unwired: 8 in]
          n218 = call "2HP_Send Cmd.vi"("Error In"=w646, "Operation"=w639, "Port"=w647) -> ("Error Out"=w644:errorcluster, "Port out"=w645:refnum<visa-resource-name>)  [unwired: 1 in]
          n219 = VISA Read(VISA resource name=w645, byte count=u32 4, error in (no error)=w644) -> (VISA resource name out=w642:refnum<visa-resource-name>, read buffer=w635:string, error out=w641:errorcluster)  [unwired: 1 out]
          n220 = call "Close serial port.vi"("Error in"=w641, "VISA resource name"=w642) -> ("Error out"=w638:errorcluster)  [unwired: 9 in]
          n221 = Reverse String(1:w635) -> (0:w636:string)
          n222 = Type Cast(type=sgl 0.0 ("byte count"), x=w636) -> (*(type *) &x=w634:sgl)
          n223 = To Unsigned Long Integer(number=w634) -> (unsigned 32bit integer=w633:u32)
          n224 = local write "Serial number"(w633) -> ()
        }
      }
    }
    frame "X" {
      # "Exit"
    }
    frame Default {
    }
  }
  "All samples out" <- w5
  "Rendezvous out" <- w1
  n225 = Merge Errors(w11, w10, w9) -> (w8:errorcluster)
  n226 = call <vilib>:"Clear Errors.vi"("error in (no error)"=w8, "specific error code to clear (0: all)"=1073676294) -> ("error out"=w16:errorcluster)  [unwired: 4 in, 1 out]
  n227 = local write "Error"(w16) -> ()
  n228 = Release Queue(queue=w15, error in (no error)=w16) -> (error out=→"Error":errorcluster)  [unwired: 1 in, 2 out]
